vi "lockin 4W simple.vi"(8 "error in (no error)":errorcluster, 10 "serial resistor":dbl=51000.0 min=0.001 max=250000.0 step=0.001 format="%.3f", 11 "VISA lockin":refnum<visa-resource-name>) -> (0 "error out":errorcluster, 1 "resistance":dbl=0.5 min=0.0 max=5.0 step=1e-06 format="%.6e", 3 "VISA session":refnum<visa-resource-name>)   [LabVIEW 2019]
panel:
  out "read buffer":string
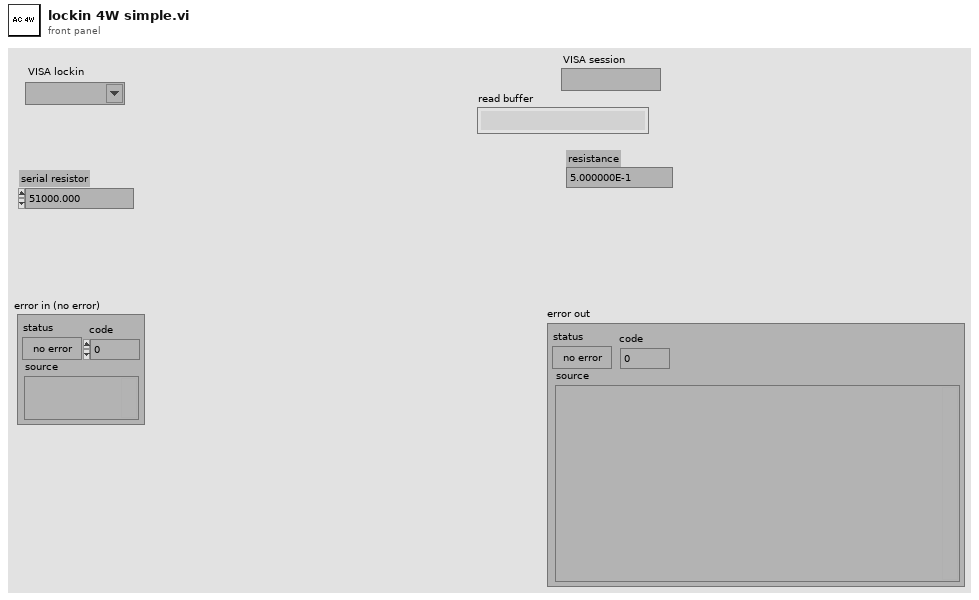
[diagram p1: front panel]
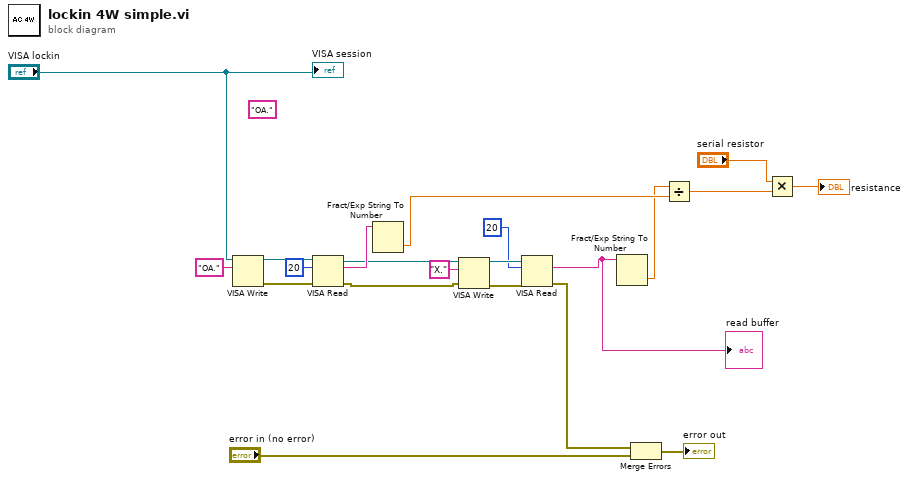
[diagram p0: block diagram]
diagram:
  (unwired) "OA." ("write buffer")
  n1 = VISA Write(VISA resource name="VISA lockin", write buffer="OA.") -> (VISA resource name out=w19:refnum<visa-resource-name>, error out=w20:errorcluster)  [unwired: 1 in, 1 out]
  n2 = VISA Read(VISA resource name=w19, byte count=u32 20, error in (no error)=w20) -> (VISA resource name out=w13:refnum<visa-resource-name>, read buffer=w18:string, error out=w6:errorcluster)  [unwired: 1 out]
  n3 = Fract/Exp String To Number(string=w18) -> (number=w17:dbl)  [unwired: 3 in, 1 out]
  n4 = VISA Write(VISA resource name=w13, write buffer="X.", error in (no error)=w6) -> (VISA resource name out=w11:refnum<visa-resource-name>, error out=w5:errorcluster)  [unwired: 1 out]
  n5 = VISA Read(VISA resource name=w11, byte count=u32 20, error in (no error)=w5) -> (read buffer=w7:string, error out=w3:errorcluster)  [unwired: 2 out]
  "read buffer" <- w7
  n6 = Fract/Exp String To Number(string=w7) -> (number=w10:dbl)  [unwired: 3 in, 1 out]
  n7 = Merge Errors(w3, "error in (no error)") -> (→"error out":errorcluster)
  n8 = Divide(x=w10, y=w17) -> (x/y=w15:dbl)
  n9 = Multiply(x="serial resistor", y=w15) -> (x*y=→"resistance":dbl)
  "VISA session" <- "VISA lockin"
